vi "Specify Process.vi"(8 "error in (no error)":errorcluster, 10 "VI Refnum":refnum<vi>, 11 "Parallel Process.lvclass in":refnum<class "Parallel Process.lvclass">) -> (0 "error out":errorcluster, 3 "Parallel Process.lvclass out":refnum<class "Parallel Process.lvclass">)   [LabVIEW 2011, in "Messenging.lvlib" / "Parallel Process.lvclass"]
uses:
  Parallel Process.lvclass
  Parallel Process.lvclass/Parallel Process.ctl
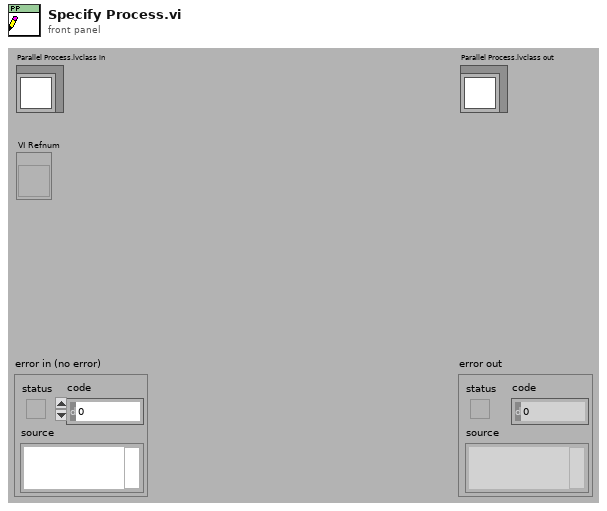
[diagram p1: front panel]
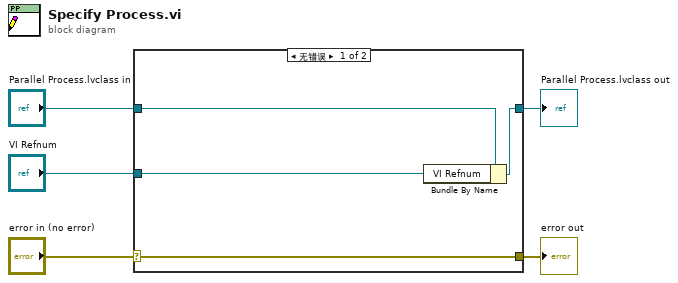
[diagram p0: block diagram]
diagram:
  n1 = case shown="无错误" "error in (no error)" {
    selector: "error in (no error)" -> [w9 w10]
    tunnel: [w9 w10] -> w4
    tunnel: [w7 w11] -> w2
    tunnel: "Parallel Process.lvclass in" -> [w8 w11]
    tunnel: "VI Refnum" -> [w6 _]
    frame No Error {
      n2 = Bundle By Name(cluster=w8, "VI Refnum"=w6) -> (w7:refnum<class "Parallel Process.lvclass">)
    }
    frame Error {
    }
  }
  "error out" <- w4
  "Parallel Process.lvclass out" <- w2
